vi "set channels.vi"(8 "error in (no error)":errorcluster, 10 "channels":refnum<class "TBM channel.lvclass">[](array[class]), 11 "module configuration in":refnum<class "tag select module configuration.lvclass">) -> (0 "error out":errorcluster, 3 "module configuration out":refnum<class "tag select module configuration.lvclass">)   [LabVIEW 2013]
uses:
  <vilib>/NI/Tag Bus Module Framework/channel/TBM channel.lvclass
  tag select module configuration.lvclass
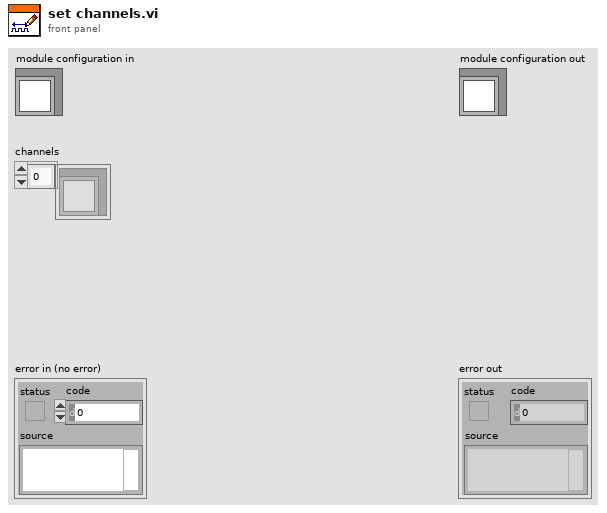
[diagram p1: front panel]
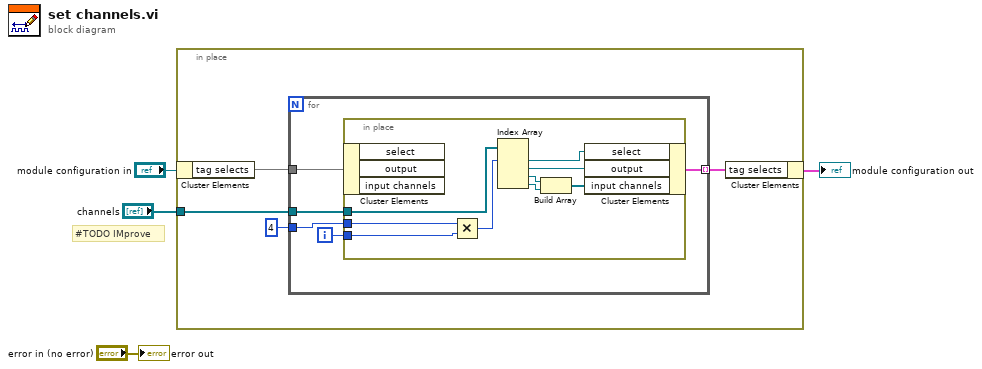
[diagram p0: block diagram]
diagram:
  # "#TODO IMprove"
  n1 = in-place {
    in-place-border: "channels" -> [w7]
    n2 = in-place-cluster #1("module configuration in") -> ("tag selects"=w8)
    n3 = for {
      tunnel: w8 -> [w10]
      tunnel: w7 -> [w13]
      tunnel: 4 -> [w11]
      tunnel: [w9] -> w5 mode=indexing
      i -> [w12]
      n4 = in-place {
        in-place-border: w13 -> [w19]
        in-place-border: w12 -> [w22]
        in-place-border: w11 -> [w21]
        n5 = in-place-cluster #2(w10) -> ()  [unwired: 3 out]
        n6 = Multiply(x=w21, y=w22) -> (x*y=w20:i32)
        n7 = Index Array(array=w19, index #1=w20) -> (element #1=w18:refnum<class "TBM channel.lvclass">, element #2=w17:refnum<class "TBM channel.lvclass">, element #3=w16:refnum<class "TBM channel.lvclass">, element #4=w15:refnum<class "TBM channel.lvclass">)  [unwired: 3 in]
        n8 = Build Array(w16, w15) -> (w14:refnum<class "TBM channel.lvclass">[])
        n9 = in-place-cluster #2("select"=w18, "output"=w17, "input channels"=w14) -> (w9:cluster{})
      }
    }
    n10 = in-place-cluster #1("tag selects"=w5) -> (→"module configuration out":cluster{})
  }
  "error out" <- "error in (no error)"
